vi "TerminateProcess.vi"(4 "error in (no error)":errorcluster, 6 "process name":string, 7 "hProcess":i32) -> (0 "error out":errorcluster, 3 "uExitCode":u32)   [LabVIEW 2011]
uses:
  KERNEL32.DLL
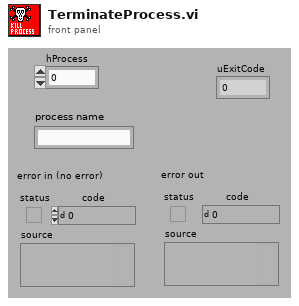
[diagram p1: front panel]
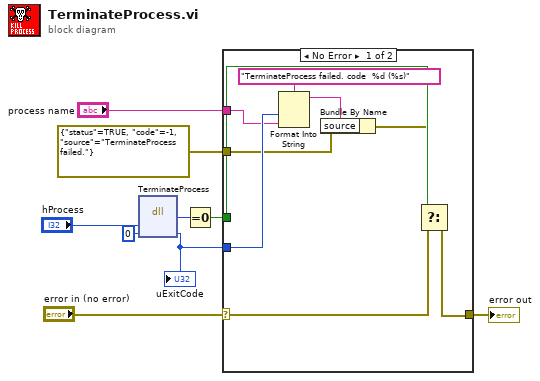
[diagram p0: block diagram]
diagram:
  n1 = dll-call lib="KERNEL32.DLL" fn="TerminateProcess"("hProcess"="hProcess", "uExitCode"=u32 0) -> (w9:i32, "uExitCode"=w3:u32)  [unwired: 4 in, 2 out]
  "uExitCode" <- w3
  n2 = Equal To 0?(x=w9) -> (x = 0?=w5:bool)
  n3 = case shown="No Error" "error in (no error)" {
    selector: "error in (no error)" -> [w17 w19]
    tunnel: [w16 w19] -> w6
    tunnel: w5 -> [w18 _]
    tunnel: w3 -> [w14 _]
    tunnel: "process name" -> [w13 _]
    tunnel: errorcluster {"status"=TRUE, "code"=-1, "source"="TerminateProcess failed."} ("error IO") -> [w12 _]
    frame No Error {
      n4 = Format Into String(format string="TerminateProcess failed. code  %d (%s)" ("source"), w14, w13) -> (resulting string=w11:string)  [unwired: 2 in, 1 out]
      n5 = Bundle By Name(cluster=w12, "source"=w11) -> (w10:errorcluster)
      n6 = Select(t=w10, s=w18, f=w17) -> (s? t:f=w16:errorcluster)
    }
    frame Error {
    }
  }
  "error out" <- w6
